vi "myRIO v1.0 Build MUX Configuration AI.vi"(11 "AI Channels List":T4) -> (3 "Channel Reservation Info":T1)   [LabVIEW 2021]
uses:
  <vilib>/myRIO/Common/Instrument Driver Framework/myRIO v1.0/AI/typedefs/AI Channels List.ctl
  <vilib>/myRIO/Common/Instrument Driver Framework/myRIO v1.0/AI/typedefs/AI Channels Enum.ctl
  <vilib>/myRIO/Common/Instrument Driver Framework/myRIO v1.0/Resource Manager/typedefs/myRIO v1.0 Channel Reservation List.ctl
  <vilib>/myRIO/Common/Instrument Driver Framework/myRIO v1.0/Resource Manager/typedefs/myRIO v1.0 Channel Reservation Info.ctl
  <vilib>/myRIO/Common/Instrument Driver Framework/myRIO v1.0/Resource Manager/typedefs/myRIO v1.0 Connector List.ctl
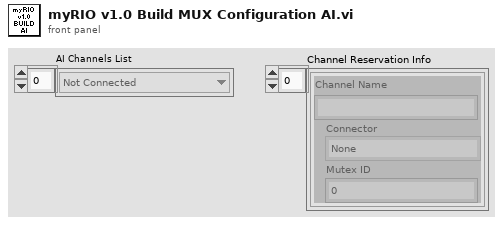
[diagram p1: front panel]
types:
  T1 = typedef "myRIO v1.0 Channel Reservation List.ctl" = T2[]
  T2 = typedef "myRIO v1.0 Channel Reservation Info.ctl" = cluster{"Channel Name":string, "Connector":T3, "Mutex ID":i32}
  T3 = typedef "myRIO v1.0 Connector List.ctl" = enum32{"None", "ConnectorA", "ConnectorB", "ConnectorC"}
  T4 = typedef "AI Channels List.ctl" = T5[]
  T5 = typedef "AI Channels Enum.ctl" = enum16{"Not Connected", "AudioIn/Left", "AudioIn/Right", "C/AI0", "C/AI1", "A/AI0", "A/AI1", "A/AI2", "A/AI3", "A/AI4", "A/AI5", "A/AI6", "A/AI7", "B/AI0", "B/AI1", "B/AI2", "B/AI3", "B/AI4", "B/AI5", "B/AI6", "B/AI7", "AI/AI0", "AI/AI1", "AI/AI2", "AI/AI3", "A/AI0 (DIFF)", "A/AI1 (DIFF)", "A/AI2 (DIFF)", "A/AI3 (DIFF)", "B/AI0 (DIFF)", "B/AI1 (DIFF)", "B/AI2 (DIFF)", "B/AI3 (DIFF)"}
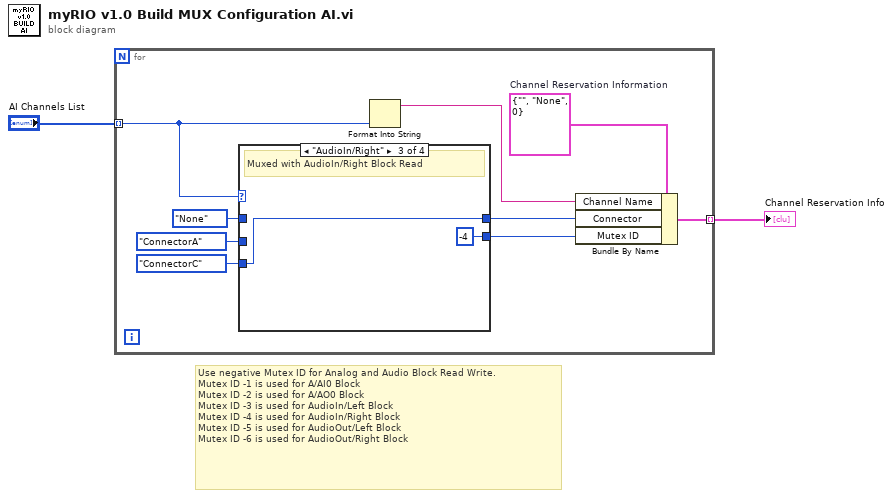
[diagram p0: block diagram]
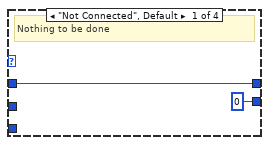
[diagram p2: hidden frame]
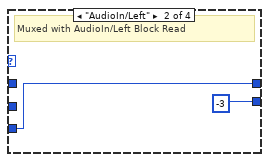
[diagram p3: hidden frame]
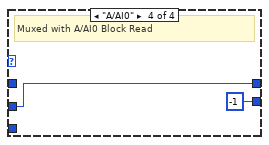
[diagram p4: hidden frame]
diagram:
  # "Use negative Mutex ID for Analog and Audio Block Read Write.\nMutex ID -1 is used for A/AI0 Block\nMutex ID -2 is used for A/AO0 Block\nMutex ID -3 is used for AudioIn/Left Block\nMutex ID -4 is used for AudioIn/Right Block\nMutex ID -5 is used for AudioOut/Left Block\nMutex ID -6 is used for AudioOut/Right Block"
  n1 = for {
    tunnel: "AI Channels List" -> [w6] mode=indexing
    tunnel: [w7] -> w1 mode=indexing
    w11 = T2 {"Channel Name"="", "Connector"=enum."None", "Mutex ID"=0}  # Channel Reservation Information
    n2 = case shown="\"AudioIn/Right\"" w6 {
      tunnel: [w13 w14 w17 w19] -> w9
      tunnel: [0 ("Bit") -3 ("Bit") -4 ("Bit") -1 ("Bit")] -> w8
      tunnel: myRIO_v1.0_Connector_List."None" ("Connector") -> [w13 _ _ _]
      tunnel: myRIO_v1.0_Connector_List."ConnectorA" ("Connector") -> [_ _ _ w19]
      tunnel: myRIO_v1.0_Connector_List."ConnectorC" ("Connector") -> [_ w14 w17 _]
      frame "Not Connected", Default {
        # "Nothing to be done"
      }
      frame "AudioIn/Left" {
        # "Muxed with AudioIn/Left Block Read"
      }
      frame "AudioIn/Right" {
        # "Muxed with AudioIn/Right Block Read"
      }
      frame "A/AI0" {
        # "Muxed with A/AI0 Block Read"
      }
    }
    n3 = Format Into String(w6) -> (resulting string=w10:string)  [unwired: 3 in, 1 out]
    n4 = Bundle By Name(cluster=w11, "Channel Name"=w10, "Connector"=w9, "Mutex ID"=w8) -> (w7:T2)
  }
  "Channel Reservation Info" <- w1
